vi "createCommandList.vi"(10 "Array":i32[](array[numeric])) -> (2 "String":string)   [LabVIEW 2013]
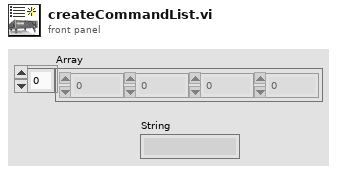
[diagram p1: front panel]
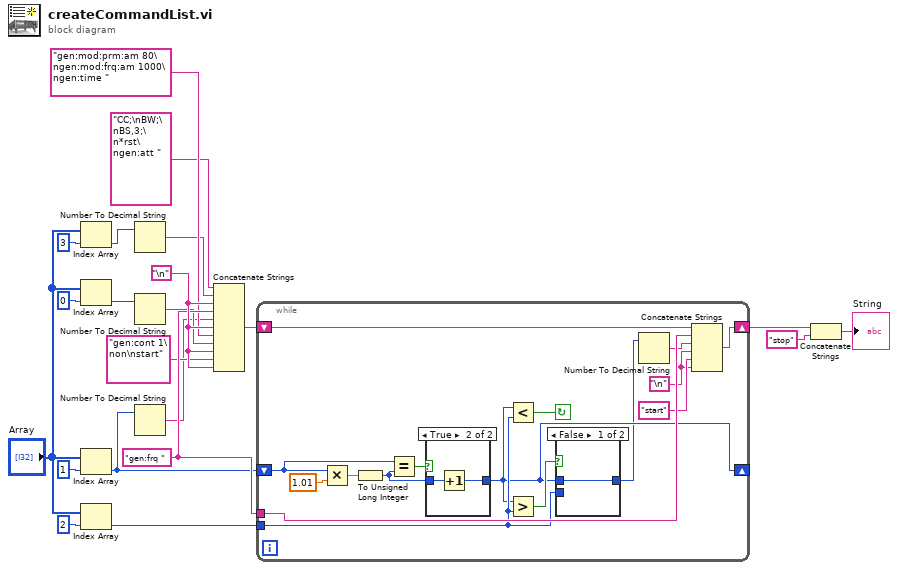
[diagram p0: block diagram]
diagram:
  w17 = "gen:frq "
  w18 = "\n"
  n1 = Index Array(array="Array", index=3) -> (element=w1:i32)
  n2 = Index Array(array="Array", index=0) -> (element=w4:i32)
  n3 = Index Array(array="Array", index=1) -> (element=w3:i32)
  n4 = Index Array(array="Array", index=2) -> (element=w2:i32)
  n5 = Number To Decimal String(number=w1) -> (decimal integer string=w11:string)  [unwired: 1 in]
  n6 = Number To Decimal String(number=w4) -> (decimal integer string=w14:string)  [unwired: 1 in]
  n7 = Number To Decimal String(number=w3) -> (decimal integer string=w12:string)  [unwired: 1 in]
  n8 = Concatenate Strings("CC;\nBW;\nBS,3;\n*rst\ngen:att ", w11, w18, w17, w12, w18, "gen:mod:prm:am 80\ngen:mod:frq:am 1000\ngen:time ", w14, w18, "gen:cont 1\non\nstart", w18) -> (w16:string)
  n9 = while {
    shift-right: [w37] -> w19
    shift-left: w16 -> [w36]
    tunnel: w17 -> [w35]
    tunnel: w2 -> [w24]
    shift-right: [w23] -> _
    shift-left: w3 -> [w26]
    stop <- w31 continue-if-true
    w32 = "\n"
    n10 = Multiply(x=w26, y=1.01) -> (x*y=w28:dbl)
    n11 = To Unsigned Long Integer(number=w28) -> (unsigned 32bit integer=w30:u32)
    n12 = Equal?(x=w26, y=w30) -> (x = y?=w29:bool)
    n13 = case shown="True" w29 {
      tunnel: w30 -> [w40 w41]
      tunnel: [w40 w42] -> w23
      frame False {
      }
      frame True {
        n14 = Increment(x=w41) -> (x+1=w42:u32)
      }
    }
    n15 = Less?(x=w23, y=w24) -> (x < y?=w31:bool)
    n16 = Greater?(x=w23, y=w24) -> (0:w25:bool)
    n17 = case shown="False" w25 {
      tunnel: w24 -> [_ w39]
      tunnel: w23 -> [w38 _]
      tunnel: [w38 w39] -> w22
      frame False {
      }
      frame True {
      }
    }
    n18 = Number To Decimal String(number=w22) -> (decimal integer string=w34:string)  [unwired: 1 in]
    n19 = Concatenate Strings(w36, w35, w34, w32, "start", w32) -> (w37:string)
  }
  n20 = Concatenate Strings(w19, "stop" ("string")) -> (→"String":string)
